vi "MALT Set One.vi"(0 "CardType":i32, 5 "Address":i32, 7 "Port":i32, 9 "State":bool, 11 "error in":errorcluster) -> (15 "error out":errorcluster)   [LabVIEW 2018]
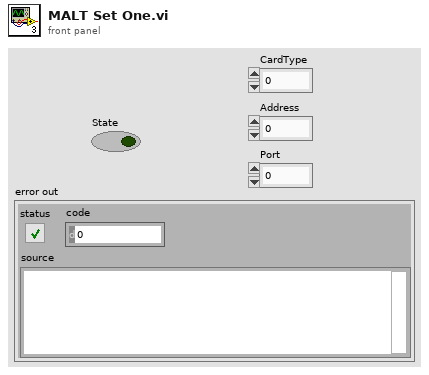
[diagram p1: front panel]
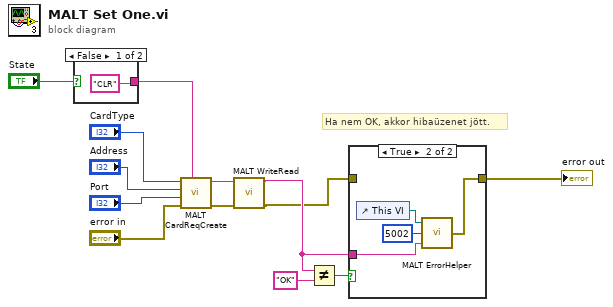
[diagram p0: block diagram]
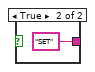
[diagram p3: hidden frame]
diagram:
  # "Ha nem OK, akkor hibaüzenet jött."
  n1 = case shown="False" "State" {
    tunnel: ["CLR" ("cmd") "SET" ("cmd")] -> w11
    frame False {
    }
    frame True {
    }
  }
  n2 = call "MALT CardReqCreate.vi"("Cmd"=w11, "error in"="error in", "Port"="Port", "Address"="Address", "CardType"="CardType") -> ("error out"=w12:errorcluster, "request"=w13:string)  [unwired: 5 in]
  n3 = call "MALT WriteRead.vi"("error in"=w12, "Request"=w13) -> ("error out"=w1:errorcluster, "Response"=w2:string)  [unwired: 8 in]
  n4 = Not Equal?(x=w2, y="OK") -> (x != y?=w4:bool)
  n5 = case shown="True" w4 {
    tunnel: w2 -> [_ w18]
    tunnel: [w16 w17] -> w3
    tunnel: w1 -> [w16 _]
    frame False {
    }
    frame True {
      n6 = control-ref of="This VI"() -> (w20:refnum<vi>)
      n7 = call "MALT ErrorHelper.vi"("Message"=w18, "Code"=5002, "This VI"=w20) -> ("error out"=w17:errorcluster)
    }
  }
  "error out" <- w3
